vi "Read separate compiled code.vi"(8 "error in (no error)":errorcluster, 11 "set source separate in":refnum<class "set source separate.lvclass">) -> (0 "error out":errorcluster, 2 "separate compiled code":bool, 3 "set source separate out":refnum<class "set source separate.lvclass">)   [LabVIEW 2013, in "set source separate.lvclass"]
uses:
  set source separate.lvclass
  set source separate.lvclass/set source separate.ctl
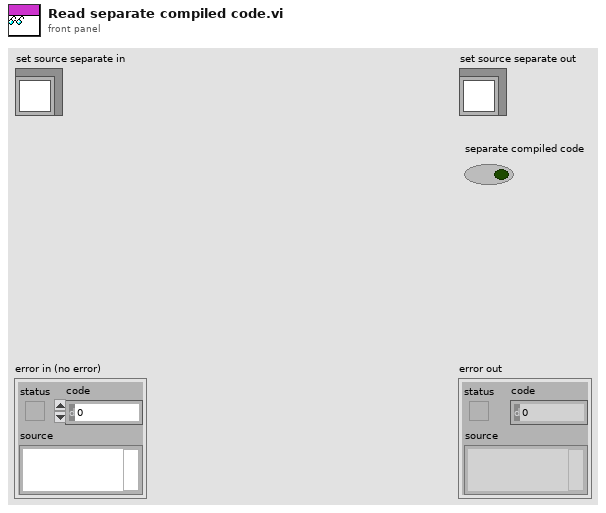
[diagram p1: front panel]
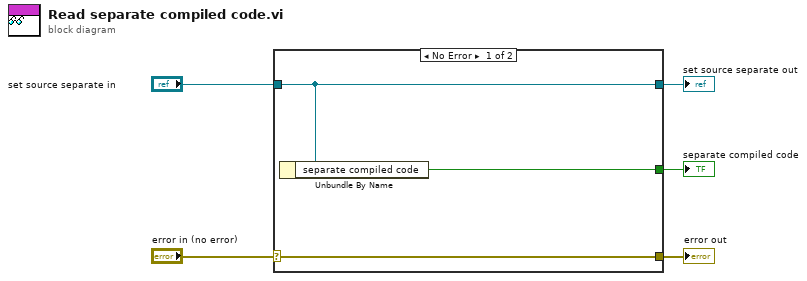
[diagram p0: block diagram]
diagram:
  n1 = case shown="No Error" "error in (no error)" {
    selector: "error in (no error)" -> [w8 w9]
    tunnel: [w8 w9] -> w4
    tunnel: [w7 w10] -> w2
    tunnel: "set source separate in" -> [w7 w10]
    tunnel: [w6 _] -> w1
    frame No Error {
      n2 = Unbundle By Name(w7) -> ("separate compiled code"=w6:bool)
    }
    frame Error {
    }
  }
  "error out" <- w4
  "set source separate out" <- w2
  "separate compiled code" <- w1
